vi "Close refs.vi"(8 "error in":errorcluster, 11 "Project":refnum<class "Project.lvclass">) -> (0 "error out":errorcluster)   [LabVIEW 2019, in "Panther Dashboard.lvlib" / "Project.lvclass"]
uses:
  Project.lvclass
  Project.lvclass/Project.ctl
  Library/Library.lvclass/Library.ctl
  Library/Read Library Ref.vi
  Read Main App Inst Ref.vi
  Read Project Ref.vi
  Read Target App Ins Ref.vi
  Read Target Ref.vi
  Read Libraries.vi
  Library/Library.lvclass
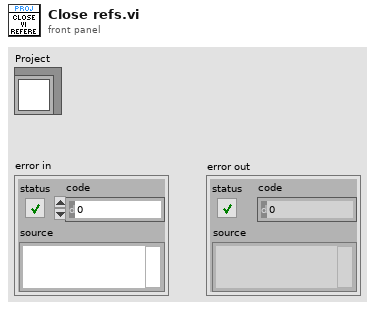
[diagram p1: front panel]
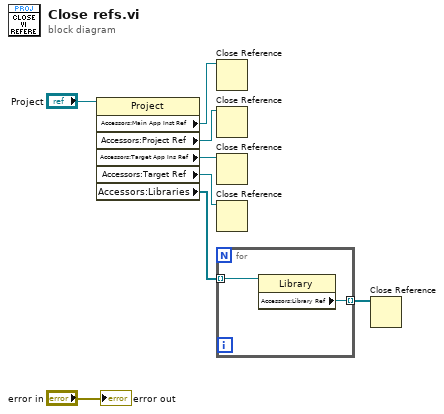
[diagram p0: block diagram]
diagram:
  n1 = property class="Project"(reference="Project") -> ("Accessors:Main App Inst Ref"=w5:refnum<vi>, "Accessors:Project Ref"=w4:refnum<vi>, "Accessors:Target App Ins Ref"=w3:refnum<vi>, "Accessors:Target Ref"=w2:refnum<vi>, "Accessors:Libraries"=w7:refnum<class "Library.lvclass">[])  [unwired: 1 in, 2 out]
  n2 = Close Reference(reference=w5) -> ()  [unwired: 1 in, 1 out]
  n3 = Close Reference(reference=w4) -> ()  [unwired: 1 in, 1 out]
  n4 = Close Reference(reference=w3) -> ()  [unwired: 1 in, 1 out]
  n5 = Close Reference(reference=w2) -> ()  [unwired: 1 in, 1 out]
  n6 = for {
    tunnel: w7 -> [w10] mode=indexing
    tunnel: [w9] -> w6 mode=indexing
    n7 = property class="Library"(reference=w10) -> ("Accessors:Library Ref"=w9:refnum<vi>)  [unwired: 1 in, 2 out]
  }
  n8 = Close Reference(reference=w6) -> ()  [unwired: 1 in, 1 out]
  "error out" <- "error in"
